vi "SECoP_dataModifyArrayLength.vi"(4 "maximum length":u32, 6 "minimum length":u32=4294967295, 7 "Position":u32, 8 "error in (no error)":errorcluster, 9 "array length":u32, 10 "SECoP_dataPtr":T1 {"ptr64" format="%.0x"; "ptr32" format="%.0x"}, 11 "DLL path (in)":T2) -> (0 "error out":errorcluster, 3 "DLL path (out)":T2)   [LabVIEW 2023, in "SECoP.lvlib"]
doc: "Call <b>\"SECoP_dataModifyArrayLength.vi\"</b> to change the length and optional the allowed minimum and maximum length of an array (SECoP_dataPtr).\n\n<b>DLL path</b> input and output of cluster from \"SECoP-Initialize.vi\"\n<b>SECoP_dataPtr</b> data to access\n<b>Position</b> points to a virtual flattened entry of the data type\n<b>array length</b> new length of the array\n<b>minimum length</b> minimum allowed length (if min<=max)\n<b>maximum length</b> maximum allowed length (if min<=max)"
uses:
  SECoP.lvlib
  SECoP-libraries.ctl
  SECoP-data.ctl
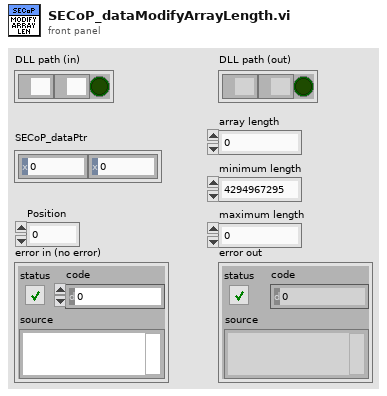
[diagram p1: front panel]
types:
  T1 = typedef "SECoP.lvlib/SECoP-data.ctl" = cluster{"ptr32":u32, "ptr64":u64}
  T2 = typedef "SECoP.lvlib/SECoP-libraries.ctl" = cluster{"serverDLL":path, "variantDLL":path, "cleanup_mode":bool}
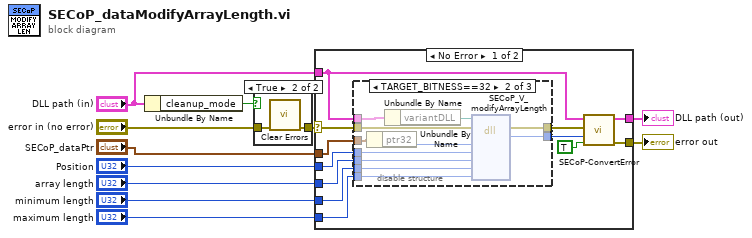
[diagram p0: block diagram]
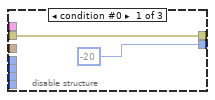
[diagram p3: hidden frame]
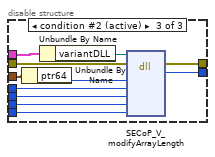
[diagram p4: hidden frame]
diagram:
  n1 = Unbundle By Name("DLL path (in)") -> ("cleanup_mode"=w8:bool)
  n2 = case shown="True" w8 {
    tunnel: "error in (no error)" -> [w12 w14]
    tunnel: [w12 w13] -> w6
    frame False {
    }
    frame True {
      n3 = call <vilib>:"Clear Errors.vi"("error in (no error)"=w14) -> ("error out"=w13:errorcluster)  [unwired: 5 in, 1 out]
    }
  }
  n4 = case shown="No Error" w6 {
    selector: w6 -> [w24 w51]
    tunnel: "DLL path (in)" -> [w15 w52]
    tunnel: [w25 w52] -> w10
    tunnel: [w26 w51] -> w9
    tunnel: "Position" -> [w20 _]
    tunnel: "SECoP_dataPtr" -> [w19 _]
    tunnel: "array length" -> [w18 _]
    tunnel: "minimum length" -> [w17 _]
    tunnel: "maximum length" -> [w16 _]
    frame No Error {
      n5 = disable-structure shown="TARGET_BITNESS==32" {
        disable-tunnel: w24 -> [w28 w39 w50]
        disable-tunnel: w15 -> [_ w38 w49]
        disable-tunnel: [w28 w37 w48] -> w23
        disable-tunnel: [-20 w36 w47] -> w22
        disable-tunnel: w20 -> [_ w35 w46]
        disable-tunnel: w19 -> [_ w33 w44]
        disable-tunnel: w18 -> [_ w32 w43]
        disable-tunnel: w17 -> [_ w31 w42]
        disable-tunnel: w16 -> [_ w30 w41]
        frame condition #0 {
        }
        frame condition #1 {
          n6 = Unbundle By Name(w33) -> ("ptr32"=w34:u32)
          n7 = Unbundle By Name(w38) -> ("variantDLL"=w29:path)
          n8 = dll-call lib="Z:/Praktische_Aufgaben/SECoP-LabVIEW2015/32bit/SECoP32.dll" fn="SECoP_V_modifyArrayLength"(path in=w29, error in=w39, "pData"=w34, "uPosition"=w35, "uLength"=w32, "uMinimumLength"=w31, "uMaximumLength"=w30) -> (error out=w37:errorcluster, "return type"=w36:i32)  [unwired: 6 in, 1 out]
        }
        frame condition #2 (active) {
          n9 = Unbundle By Name(w44) -> ("ptr64"=w45:u64)
          n10 = Unbundle By Name(w49) -> ("variantDLL"=w40:path)
          n11 = dll-call lib="Z:/Praktische_Aufgaben/SECoP-LabVIEW2015/32bit/SECoP32.dll" fn="SECoP_V_modifyArrayLength"(path in=w40, error in=w50, "pData"=w45, "uPosition"=w46, "uLength"=w43, "uMinimumLength"=w42, "uMaximumLength"=w41) -> (error out=w48:errorcluster, "return type"=w47:i32)  [unwired: 6 in, 1 out]
        }
      }
      n12 = call "SECoP-ConvertError.vi"("return is boolean"=TRUE, "return code"=w22, "error in (no error)"=w23, "DLL path (in)"=w15) -> ("error out"=w26:errorcluster, "DLL path (out)"=w25:T2)  [unwired: 6 in]
    }
    frame Error {
    }
  }
  "DLL path (out)" <- w10
  "error out" <- w9
